vi "ConfigArbWfrm.vi"(8 "error in (no error)":errorcluster, 11 "ClassIn":refnum<class "NISTFGenPluginsBase.lvclass">) -> (0 "error out":errorcluster, 3 "ClassOut":refnum<class "NISTFGenPluginsBase.lvclass">)   [LabVIEW 2014, in "FGenPlugins.lvlib" / "NISTFGenPluginsBase.lvclass"]
uses:
  NISTFGenPluginsBase.lvclass
  <userlib>/NIST/BaseClasses/Object_class/BaseObject.lvclass
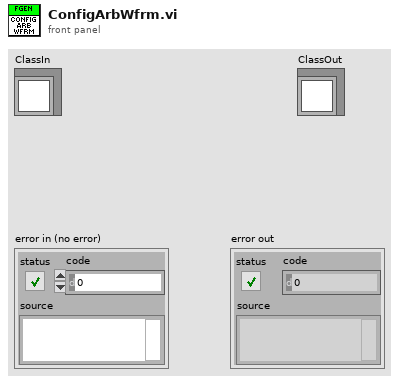
[diagram p1: front panel]
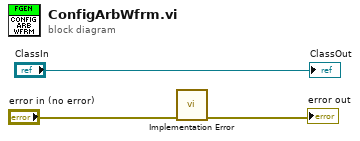
[diagram p0: block diagram]
diagram:
  n1 = call <userlib>:"Implementation Error.vi"("error in (no error)"="error in (no error)") -> ("error out"=→"error out":errorcluster)  [unwired: 10 in]
  "ClassOut" <- "ClassIn"
